vi "set_lc_sp.vi"(6 "yw":string, 8 "sp_shuoming":string, 9 "sp_yijian":string, 10 "id":string, 11 "lc_num":string) -> (1 "cur_spnum":string, 3 "cur_spsta":string, 5 "fqren":string)   [LabVIEW 2017, in "Lib_code.lvlib"]
uses:
  Lib_code.lvlib
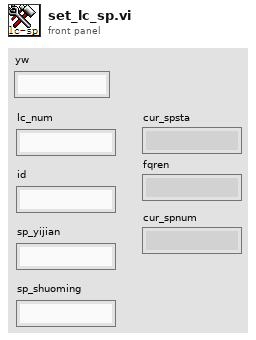
[diagram p1: front panel]
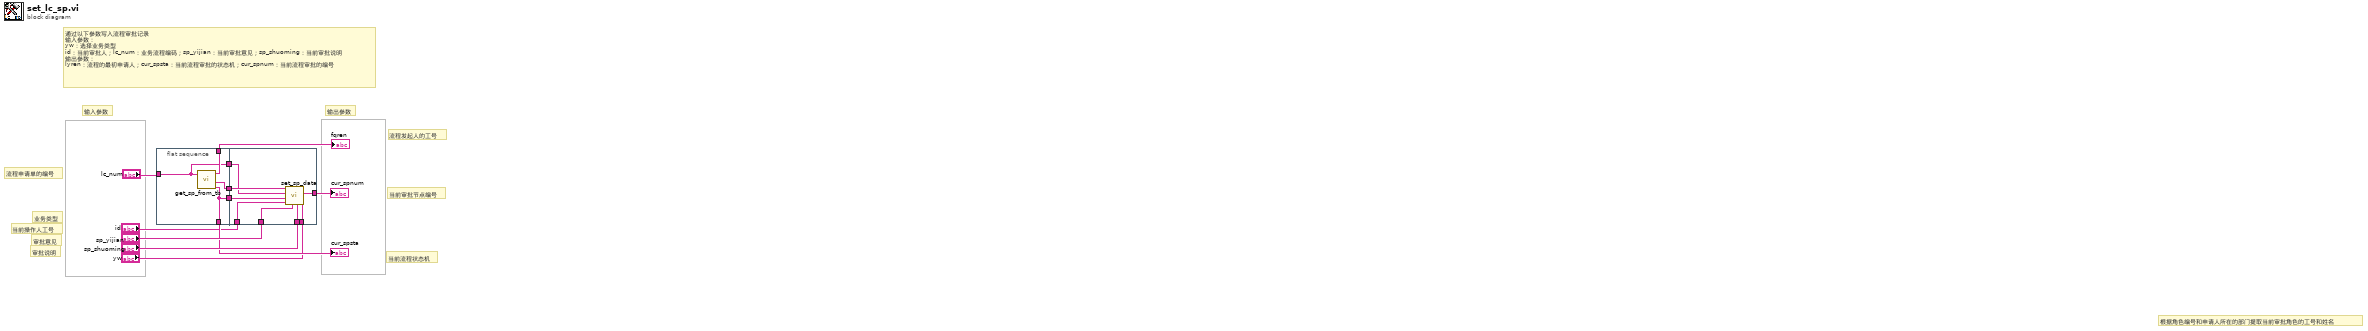
[diagram p0: block diagram]
diagram:
  # "当前审批节点编号"
  # "当前流程状态机"
  # "流程发起人的工号"
  # "输出参数"
  # "审批说明"
  # "审批意见"
  # "当前操作人工号"
  # "业务类型"
  # "流程申请单的编号"
  # "输入参数"
  # "通过以下参数写入流程审批记录\n输入参数：\nyw：选择业务类型\nid：当前审批人；lc_num：业务流程编码；sp_yijian：当前审批意见；sp_shuoming：当前审批说明\n输出参数：\nlyren：流程的最初申请人；cur_spsta：当前流程审批的状态机；cur_spnum：当前流程审批的编号"
  # "根据角色编号和申请人所在的部门提取当前审批角色的工号和姓名"
  n1 = flat-sequence {
    tunnel: "lc_num" -> [w13]
    tunnel: [w15] -> w6
    tunnel: [w14] -> w4
    tunnel: [w12] -> w3
    tunnel: [w13] -> w2
    tunnel: [w12] -> w8
    tunnel: [w23] -> w5
    tunnel: w4 -> [w22]
    tunnel: w3 -> [w21]
    tunnel: "id" -> [w20]
    tunnel: "sp_yijian" -> [w19]
    tunnel: "sp_shuoming" -> [w18]
    tunnel: w2 -> [w17]
    tunnel: "yw" -> [w16]
    frame #0 {
      n2 = call "get_sp_from_tb.vi"("lc_num"=w13) -> ("nx_spsta"=w12:string, "cur_spnum"=w14:string, "fqren"=w15:string)  [unwired: 3 in, 1 out]
    }
    frame #1 {
      n3 = call "set_sp_data.vi"("yw"=w16, "sp_shuoming"=w18, "sp_yijian"=w19, "sp_ren"=w20, "cur_spsta"=w21, "lc_num"=w17, "pro_spnum"=w22) -> ("spnum"=w23:string)  [unwired: 3 in, 1 out]
    }
  }
  "cur_spnum" <- w5
  "fqren" <- w6
  "cur_spsta" <- w8
